vi "DrawFormattedString.vi"(0 "reference":refnum<class "MultiLineString.lvclass">, 1 "graphics":refnum<class "Graphics.lvclass">, 2 "bounds":T1 {"height" format="%.2f"; "width" format="%.2f"; "y" format="%.2f"; "x" format="%.2f"}, 5 "error in (no error)":errorcluster) -> (14 "reference out":refnum<class "MultiLineString.lvclass">, 19 "error out":errorcluster)   [LabVIEW 2012, in "MultiLineString.lvclass"]
doc: "public void draw(Graphics2D g2, Rectangle2D r)"
uses:
  <resource>/Framework/Providers/Open_GDS/UML/MultiLineString_class/MultiLineString.lvclass
  <resource>/Framework/Providers/Open_GDS/UML/Graphics_class/Graphics.lvclass
  <resource>/Framework/Providers/Open_GDS/UML/General/Rectangle/Rectangle Rectangle2D.ctl
  <resource>/Framework/Providers/Open_GDS/UML/General/Point/Point Point2D.ctl
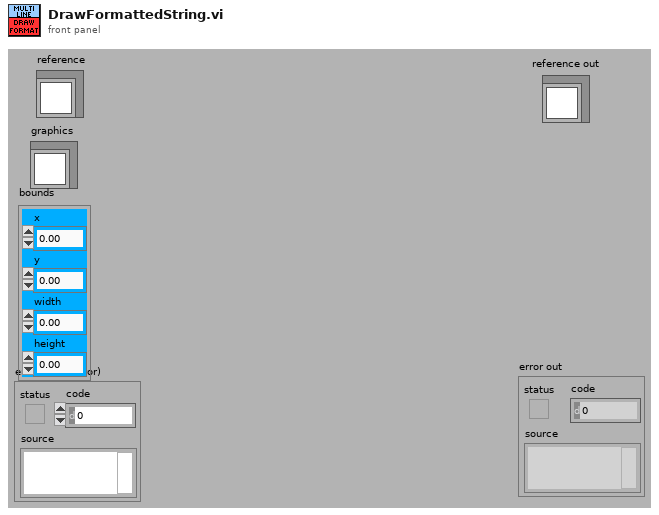
[diagram p1: front panel]
types:
  T1 = typedef "Rectangle Rectangle2D.ctl" = cluster{"x":dbl, "y":dbl, "width":dbl, "height":dbl}
  T2 = typedef "Point Point2D.ctl" = cluster{"x":dbl, "y":dbl}
  T3 = typedef "MultiLineString.lvclass/ObjectAttributes.ctl" = cluster{"GAP":i32, "text":string, "justification":T4, "size":T5, "underlined":bool}
  T4 = typedef "MultiLineString.lvclass/JustificationType.ctl" = enum16{"LEFT", "CENTER", "RIGHT"}
  T5 = typedef "MultiLineString.lvclass/SizeType.ctl" = enum16{"LARGE", "NORMAL", "SMALL"}
  T6 = typedef "Graphics.lvclass/LvFontType.ctl" = enum16{"User-specified Font", "Application Font", "System Font", "Dialog Font"}
  T7 = typedef "Graphics.lvclass/FontType.ctl" = cluster{"Font Name:":string, "Size":i16, "Strikeout?":bool, "Italic?":bool, "Underline?":bool, "Outline?":bool, "Shadow?":bool, "Bold?":bool}
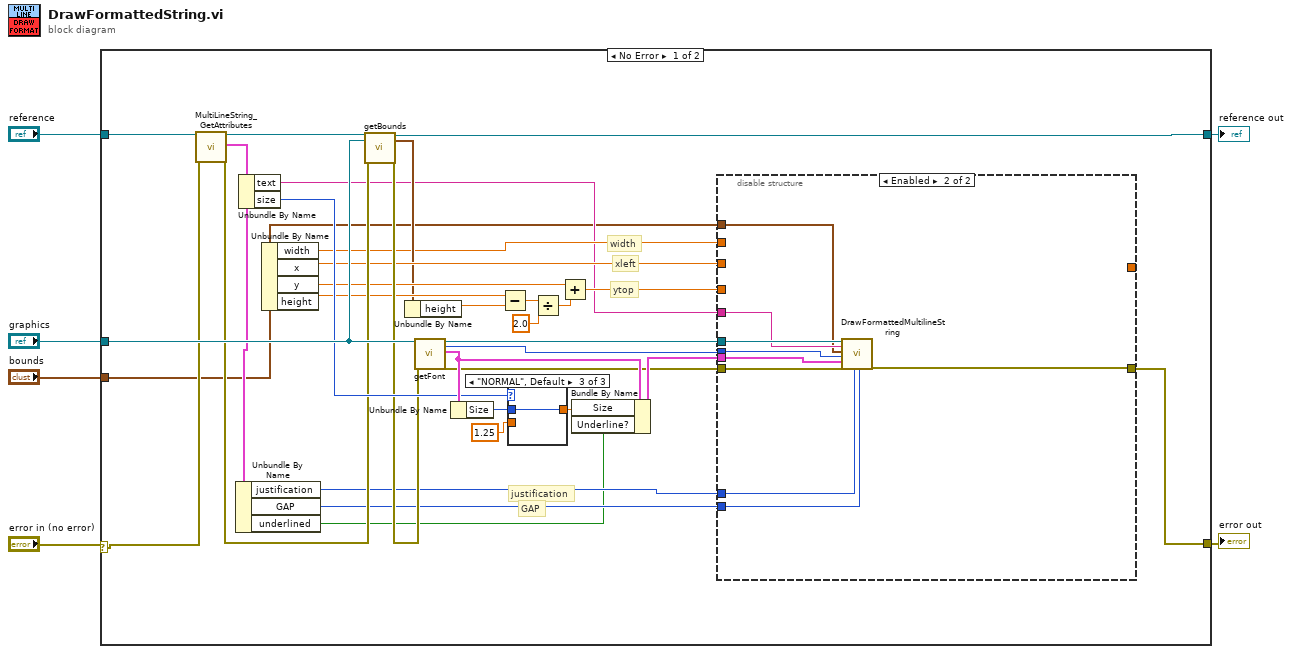
[diagram p0: block diagram]
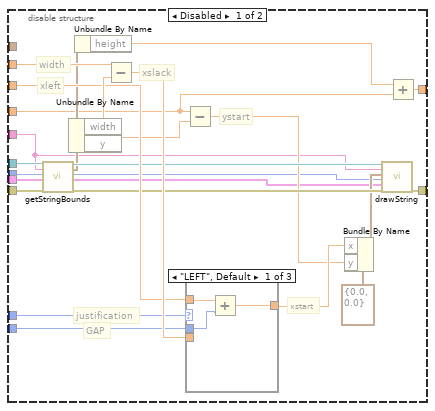
[diagram p2: hidden frame]
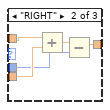
[diagram p3: hidden frame]
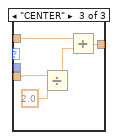
[diagram p4: hidden frame]
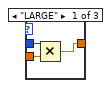
[diagram p5: hidden frame]
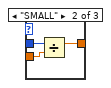
[diagram p6: hidden frame]
diagram:
  n1 = case shown="No Error" "error in (no error)" {
    selector: "error in (no error)" -> [w35 w92]
    tunnel: "reference" -> [w39 w93]
    tunnel: [w38 w92] -> w5
    tunnel: [w37 w93] -> w4
    tunnel: "graphics" -> [w36 _]
    tunnel: "bounds" -> [w7 _]
    frame No Error {
      # "GAP"
      # "justification"
      # "width"
      # "xleft"
      # "ytop"
      n2 = call <resource>:"MultiLineString_GetAttributes.vi"("reference in"=w39, "error in (no error)"=w35) -> ("reference out"=w34:refnum<class "MultiLineString.lvclass">, "Attributes"=w13:T3, "error out"=w24:errorcluster)  [unwired: 15 out]
      n3 = Unbundle By Name(w13) -> ("justification"=w12:T4, "GAP"=w11:i32, "underlined"=w10:bool)
      n4 = Unbundle By Name(w13) -> ("text"=w8:string, "size"=w25:T5)
      n5 = Unbundle By Name(w7) -> ("width"=w14:dbl, "x"=w21:dbl, "y"=w22:dbl, "height"=w20:dbl)
      n6 = call-dynamic "getBounds.vi"("reference"=w34, "graphics"=w36, "error in (no error)"=w24) -> ("reference out"=w37:refnum<class "MultiLineString.lvclass">, "bounds"=w19:T1, "error out"=w23:errorcluster)  [unwired: 14 out]
      n7 = Unbundle By Name(w19) -> ("height"=w18:dbl)
      n8 = call <resource>:"getFont.vi"("reference"=w36, "error in (no error)"=w23) -> ("reference out"=w33:refnum<class "Graphics.lvclass">, "fontType"=w32:T6, "font"=w29:T7, "error out"=w26:errorcluster)  [unwired: 14 out]
      n9 = Unbundle By Name(w29) -> ("Size"=w31:i16)
      n10 = Subtract(x=w20, y=w18) -> (x-y=w17:dbl)
      n11 = case shown="\"NORMAL\", Default" w25 {
        tunnel: w31 -> [w87 w89 w91]
        tunnel: 1.25 ("y") -> [w86 w90 _]
        tunnel: [w85 w88 w91] -> w27
        frame "LARGE" {
          n12 = Multiply(x=w87, y=w86) -> (x*y=w85:dbl)
        }
        frame "SMALL" {
          n13 = Divide(x=w89, y=w90) -> (x/y=w88:dbl)
        }
        frame "NORMAL", Default {
        }
      }
      n14 = Divide(x=w17, y=2.0) -> (x/y=w16:dbl)
      n15 = Add(x=w22, y=w16) -> (x+y=w9:dbl)
      n16 = Bundle By Name(cluster=w29, "Size"=w27, "Underline?"=w10) -> (w28:T7)
      n17 = disable-structure shown="Enabled" {
        disable-tunnel: w14 -> [w62 _]
        disable-tunnel: w21 -> [w59 _]
        disable-tunnel: [w55 w79] -> w38
        disable-tunnel: [w50 _] -> _
        disable-tunnel: w9 -> [w47 _]
        disable-tunnel: w33 -> [w46 w84]
        disable-tunnel: w8 -> [w45 w83]
        disable-tunnel: w32 -> [w44 w77]
        disable-tunnel: w28 -> [w43 w78]
        disable-tunnel: w26 -> [w42 w82]
        disable-tunnel: w12 -> [w41 w81]
        disable-tunnel: w11 -> [w40 w80]
        disable-tunnel: w7 -> [_ w76]
        frame Disabled {
          # "ystart"
          # "xstart"
          # "xleft"
          # "width"
          # "justification"
          # "GAP"
          # "xslack"
          n18 = call-dynamic "getStringBounds.vi"("reference"=w46, "text"=w45, "fontType"=w44, "font"=w43, "error in (no error)"=w42) -> ("reference out"=w57:refnum<class "Graphics.lvclass">, "bounds"=w49:T1, "error out"=w56:errorcluster)  [unwired: 12 out]
          n19 = Unbundle By Name(w49) -> ("width"=w61:dbl, "y"=w58:dbl)
          n20 = Unbundle By Name(w49) -> ("height"=w48:dbl)
          n21 = Subtract(x=w62, y=w61) -> (x-y=w60:dbl)
          n22 = Subtract(x=w47, y=w58) -> (x-y=w51:dbl)
          n23 = case shown="\"LEFT\", Default" w41 {
            tunnel: w60 -> [_ w69 w74]
            tunnel: w59 -> [w65 w70 w72]
            tunnel: w40 -> [w64 w67 _]
            tunnel: [w63 w66 w71] -> w52
            frame "LEFT", Default {
              n24 = Add(x=w65, y=w64) -> (x+y=w63:dbl)
            }
            frame "RIGHT" {
              n25 = Add(x=w70, y=w69) -> (x+y=w68:dbl)
              n26 = Subtract(x=w68, y=w67) -> (x-y=w66:dbl)
            }
            frame "CENTER" {
              n27 = Divide(x=w74, y=2.0) -> (x/y=w73:dbl)
              n28 = Add(x=w72, y=w73) -> (x+y=w71:dbl)
            }
          }
          n29 = Bundle By Name(cluster=T2 {"x"=0.0, "y"=0.0} ("textPos"), "x"=w52, "y"=w51) -> (w53:T2)
          n30 = call-dynamic "drawString.vi"("reference"=w57, "text"=w45, "textPos"=w53, "fontType"=w44, "font"=w43, "error in (no error)"=w56) -> ("error out"=w55:errorcluster)  [unwired: 1 in, 12 out]
          n31 = Add(x=w48, y=w47) -> (x+y=w50:dbl)
        }
        frame Enabled {
          n32 = call-dynamic "DrawFormattedMultilineString.vi"("reference"=w84, "text"=w83, "bounds"=w76, "fontType"=w77, "font"=w78, "error in (no error)"=w82, "Justification"=w81, "GAP"=w80) -> ("error out"=w79:errorcluster)  [unwired: 10 in, 1 out]
        }
      }
    }
    frame Error {
    }
  }
  "reference out" <- w4
  "error out" <- w5
